vi "wait_non_blocking.vi"(0 "Error in":errorcluster, 1 "Seconds to wait":i32) -> ()   [LabVIEW 2015]
doc: "Waits for the given number of seconds, stopping partway if a stop notification is received through the queue. This is helpful when you want to delay in a loop but don't want to make the program unresponsive to stop commands."
uses:
  Signaller/Signaller.lvclass
panel:
  in  "Stop signaller":refnum<class "Signaller.lvclass">
  out "Error out":errorcluster
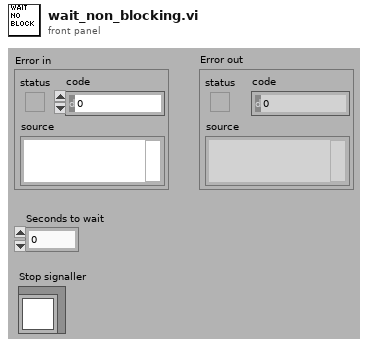
[diagram p1: front panel]
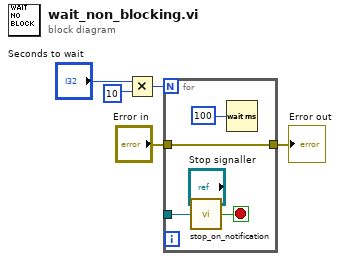
[diagram p0: block diagram]
diagram:
  n1 = Multiply(x="Seconds to wait", y=10) -> (x*y=w1:i32)
  n2 = for {
    N: w1 -> [_]
    tunnel: [w8] -> w5
    tunnel: "Error in" -> [w7]
    tunnel: [w7] -> w4
    stop <- w9 stop-if-true
    n3 = call "stop_on_notification.vi"("Notofication queue"=w8) -> ("Should stop"=w9:bool)
    n4 = Wait (ms)(milliseconds to wait=u32 100) -> ()  [unwired: 1 out]
  }
  "Error out" <- w4
